vi "LoadScript.vi"() -> ()   [LabVIEW 2012]
uses:
  <vilib>/regexp/Match Regular Expression.xnode
panel:
  in  "Script":path
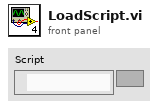
[diagram p1: front panel]
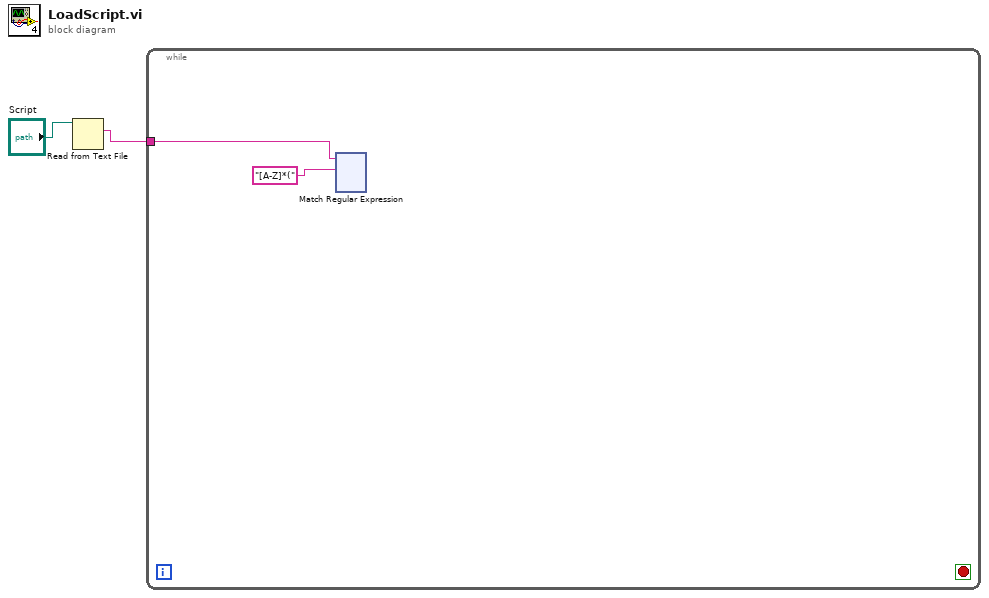
[diagram p0: block diagram]
diagram:
  n1 = Read from Text File(file (use dialog)="Script") -> (text=w1:string)  [unwired: 3 in, 3 out]
  n2 = while {
    tunnel: w1 -> [w3]
    stop <- _ stop-if-true
    n3 = xnode "Match Regular Expression"("input string"=w3, "regular expression"="[A-Z]*(") -> ()  [unwired: 4 in, 5 out]
  }
